vi "Read Report.vi"(8 "error in (no error)":errorcluster, 11 "Report Generator in":refnum<class "Report Generator.lvclass">) -> (0 "error out":errorcluster, 2 "Report.lvlibp:Report.lvclass":refnum<class "Report.lvclass">, 3 "Report Generator out":refnum<class "Report Generator.lvclass">)   [LabVIEW 2023, in "Report Generator.lvlib" / "Report Generator.lvclass"]
uses:
  Library/Report Generator.lvclass
  builds/Tools/Report.lvlibp/Report.lvclass
  Library/Report Generator.lvclass/Report Generator.ctl
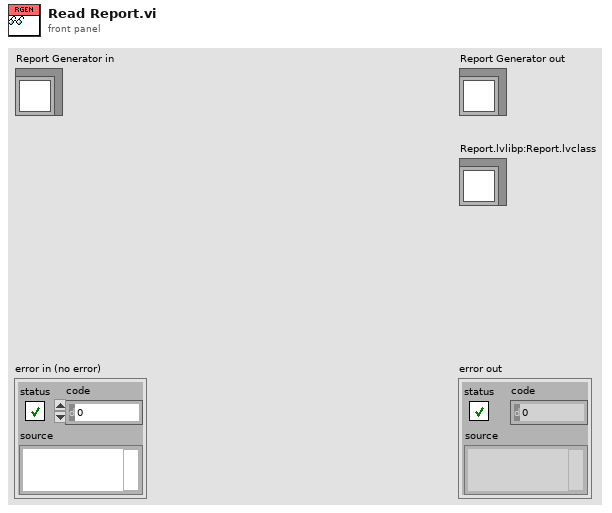
[diagram p1: front panel]
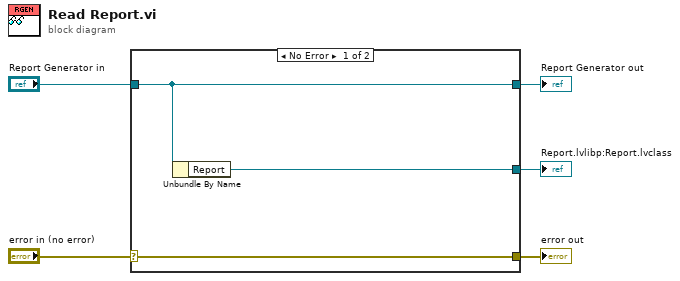
[diagram p0: block diagram]
diagram:
  n1 = case shown="No Error" "error in (no error)" {
    selector: "error in (no error)" -> [w8 w9]
    tunnel: [w8 w9] -> w4
    tunnel: [w7 w10] -> w2
    tunnel: "Report Generator in" -> [w7 w10]
    tunnel: [w6 _] -> w1
    frame No Error {
      n2 = Unbundle By Name(w7) -> ("Report"=w6:refnum<class "Report.lvclass">)
    }
    frame Error {
    }
  }
  "error out" <- w4
  "Report Generator out" <- w2
  "Report.lvlibp:Report.lvclass" <- w1
